vi "Images FG.vi"(10 "All Images In":T1[](array[typedef]), 11 "Image":T2) -> (3 "Flattened Image":T1)   [LabVIEW 2020, in "TSnax UI.lvlib"]
uses:
  TSnax UI.lvlib
  Image.ctl
  <vilib>/picture/picture.llb/imagedata.ctl
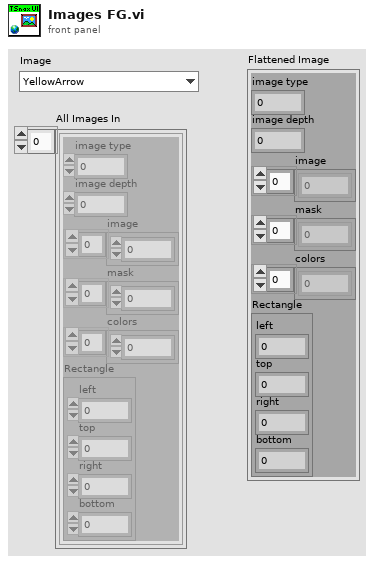
[diagram p1: front panel]
types:
  T1 = typedef "imagedata.ctl" = cluster{"image type":i32, "image depth":i32, "image":u8[], "mask":u8[], "colors":u32[], "Rectangle":cluster{"left":i16, "top":i16, "right":i16, "bottom":i16}}
  T2 = typedef "TSnax UI.lvlib/Image.ctl" = enum16{"YellowArrow", "GreenArrow"}
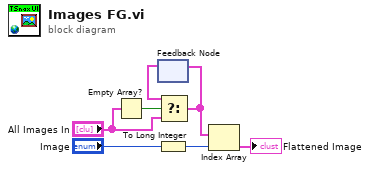
[diagram p0: block diagram]
diagram:
  n1 = Empty Array?(array="All Images In") -> (empty?=w7:bool)
  n2 = feedback #1() -> (w5:T1[])  [unwired: 1 in]
  n3 = To Long Integer(number="Image") -> (32bit integer=w3:i32)
  n4 = Select(t=w5, s=w7, f="All Images In") -> (s? t:f=w4:T1[])
  n5 = feedback-in #1(w4) -> ()
  n6 = Index Array(array=w4, index=w3) -> (element=→"Flattened Image":T1)
